vi "Blend.vi"(7 "Source Name in":string, 8 "error in (no error)":errorcluster, 9 "Source Enqueuer":refnum<class "Message Enqueuer.lvclass">, 10 "Sample to Blend in":refnum<class "Sample.lvclass">, 11 "CO2 Actor in":refnum<class "CO2 Actor.lvclass">) -> (0 "error out":errorcluster, 2 "Source Name":string, 3 "CO2 Actor out":refnum<class "CO2 Actor.lvclass">)   [LabVIEW 2015, in "cRIO-Carbondioxide.lvlib" / "CO2-Actor.lvlib" / "CO2 Actor.lvclass"]
uses:
  CO2 Actor.lvclass
  subs/Sample/Sample.lvclass
  <vilib>/ActorFramework/Message Enqueuer/Message Enqueuer.lvclass
  subs/Sample/Sample.lvclass/Sample.ctl
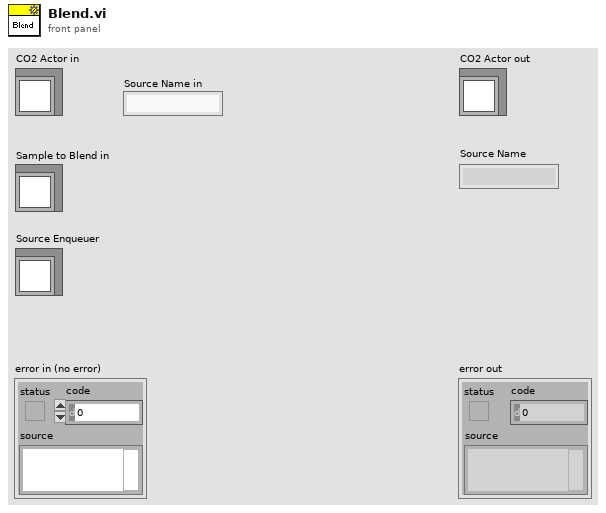
[diagram p1: front panel]
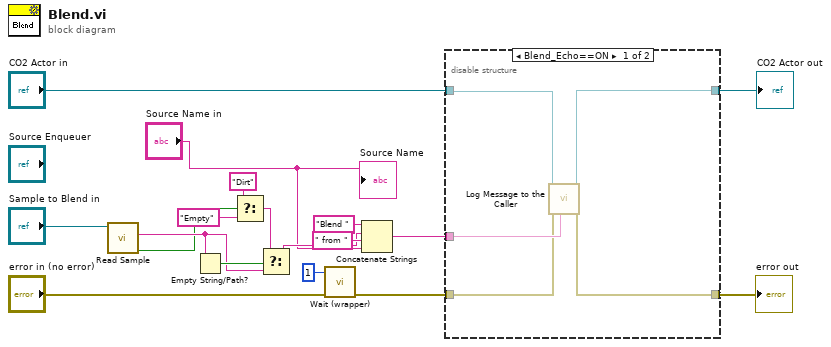
[diagram p0: block diagram]
diagram:
  n1 = call "Read Sample.vi"("Sample in"="Sample to Blend in") -> ("Sample In"=w7:bool, "Name"=w11:string)  [unwired: 6 in, 3 out]
  n2 = Empty String/Path?(string/path=w11) -> (empty?=w12:bool)
  n3 = Select(t="Dirt", s=w7, f="Empty") -> (s? t:f=w5:string)
  n4 = Select(t=w5, s=w12, f=w11) -> (s? t:f=w10:string)
  n5 = call "Wait (wrapper).vi"("milliseconds to wait (200)"=u32 1, "error in (no error)"="error in (no error)") -> ("error out"=w2:errorcluster)  [unwired: 9 in]
  n6 = Concatenate Strings("Blend " ("String (\"OK\")"), w10, " from " ("string"), "Source Name in") -> (w14:string)
  n7 = disable-structure shown="Blend_Echo==ON" {
    disable-tunnel: "CO2 Actor in" -> [w22 w24]
    disable-tunnel: [w21 w24] -> w15
    disable-tunnel: w14 -> [w23 _]
    disable-tunnel: [w20 w25] -> w4
    disable-tunnel: w2 -> [w19 w25]
    frame condition #0 {
      n8 = call-dynamic "Log Message to the Caller.vi"("String (\"\" = no message to send)"=w23, "error in (no error)"=w19, "CO2 Actor in"=w22) -> ("error out"=w20:errorcluster, "CO2 Actor out"=w21:refnum<class "CO2 Actor.lvclass">)  [unwired: 7 in]
    }
    frame condition #1 (active) {
    }
  }
  "error out" <- w4
  "CO2 Actor out" <- w15
  "Source Name" <- "Source Name in"
